vi "2-FindMsgs.vi"(3 "ProjectIndex":i32) -> (1 "Project-Name":string)   [LabVIEW 2014, in "TestVIs.lvlib"]
uses:
  TestVIs.lvlib
panel:
  out "Messages":T1(array[cluster])
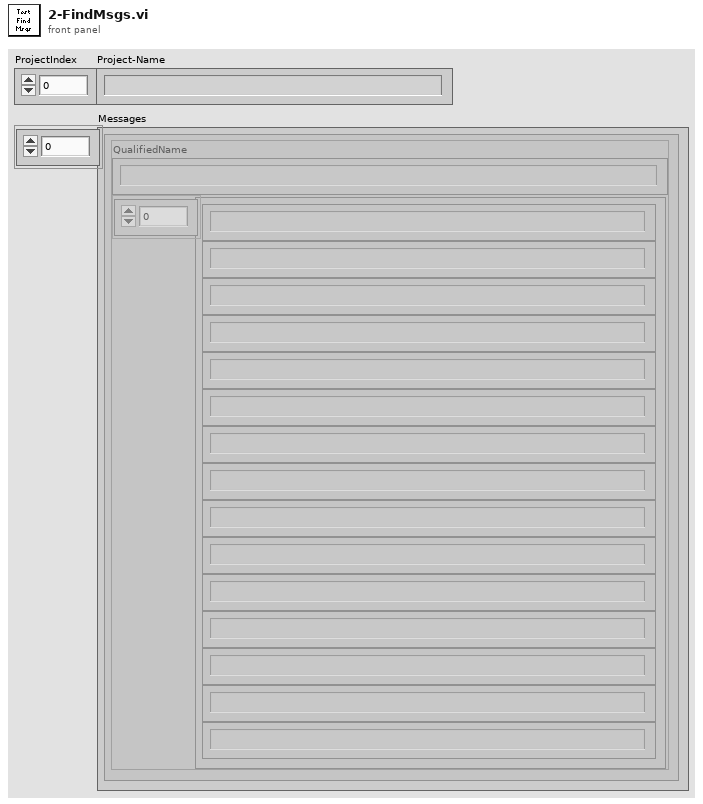
[diagram p1: front panel]
types:
  T1 = cluster{"QualifiedName":string, "Array":string[]}[]
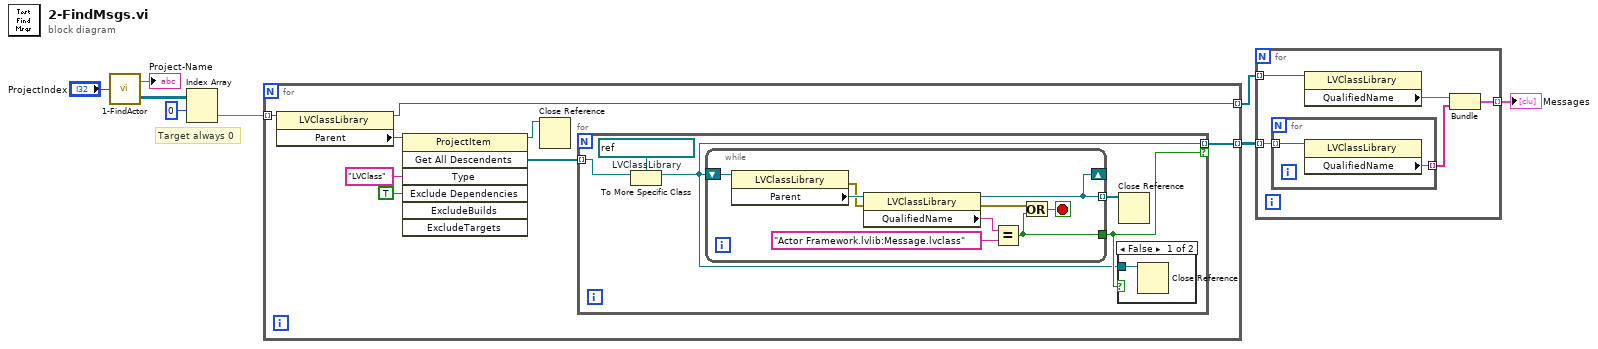
[diagram p0: block diagram]
diagram:
  # "Target always 0"
  n1 = call "1-FindActor.vi"("ProjectIndex"="ProjectIndex") -> ("Actors"=w6:refnum<vi>[][], "Project-Name"=→"Project-Name":string)  [unwired: 2 in]
  n2 = Index Array(array=w6, index (row)=0) -> (element=w4:refnum<vi>[])  [unwired: 1 in]
  n3 = for {
    tunnel: w4 -> [w10] mode=indexing
    tunnel: [w11] -> w3 mode=indexing
    tunnel: [w9] -> w2 mode=indexing
    n4 = property class="LVClassLibrary"(reference=w10) -> (reference out=w9:refnum<vi>, "Parent"=w13:refnum<vi>)  [unwired: 1 in, 1 out]
    n5 = invoke class="ProjectItem" method="Get All Descendents"(reference=w13, "Type"="LVClass", "Exclude Dependencies"=TRUE ("ExcludeDependencies")) -> (reference out=w14:refnum<vi>, "All Descendents"=w12:refnum<vi>[])  [unwired: 4 in, 5 out]
    n6 = Close Reference(reference=w14) -> ()  [unwired: 1 in, 1 out]
    n7 = for {
      tunnel: w12 -> [w20] mode=indexing
      tunnel: [w17] -> w11 mode=indexing if=w18
      w21 = refnum<vi> refnum  # LVClassLibrary
      n8 = To More Specific Class(target class=w21, reference=w20) -> (specific class reference=w17:refnum<vi>)  [unwired: 1 in, 1 out]
      n9 = while {
        shift-right: [w25] -> _
        shift-left: w17 -> [w31]
        tunnel: [w25] -> w19 mode=indexing
        tunnel: [w24] -> w18
        stop <- w26 stop-if-true
        n10 = property class="LVClassLibrary"(reference=w31) -> (error out=w23:errorcluster, "Parent"=w27:refnum<vi>)  [unwired: 1 in, 1 out]
        n11 = property class="LVClassLibrary"(reference=w27, error in=w23) -> (reference out=w25:refnum<vi>, error out=w28:errorcluster, "QualifiedName"=w30:string)
        n12 = Equal?(x=w30, y="Actor Framework.lvlib:Message.lvclass") -> (x = y?=w24:bool)
        n13 = Or(x=w28, y=w24) -> (x .or. y?=w26:bool)
      }
      n14 = case shown="False" w18 {
        tunnel: w17 -> [w22 _]
        frame False {
          n15 = Close Reference(reference=w22) -> ()  [unwired: 1 in, 1 out]
        }
        frame True {
        }
      }
      n16 = Close Reference(reference=w19) -> ()  [unwired: 1 in, 1 out]
    }
  }
  n17 = for {
    tunnel: w3 -> [w36] mode=indexing
    tunnel: w2 -> [w35] mode=indexing
    tunnel: [w32] -> w1 mode=indexing
    n18 = for {
      tunnel: w36 -> [w38] mode=indexing
      tunnel: [w37] -> w33 mode=indexing
      n19 = property class="LVClassLibrary"(reference=w38) -> ("QualifiedName"=w37:string)  [unwired: 1 in, 2 out]
    }
    n20 = property class="LVClassLibrary"(reference=w35) -> ("QualifiedName"=w34:string)  [unwired: 1 in, 2 out]
    n21 = Bundle("QualifiedName"=w34, w33) -> (w32:cluster{"QualifiedName":string, string[]})  [unwired: 1 in]
  }
  "Messages" <- w1
